vi "文本文件（将100个正弦数据以3位小数的形式写入文本文件的尾部）.vi"() -> ()   [LabVIEW 2017]
panel:
  out "写入数据":dbl[](array[numeric])
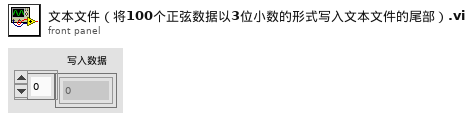
[diagram p1: front panel]
types:
  T1 = enum16{"open", "replace", "create", "open or create", "replace or create", "replace or create with confirmation"}
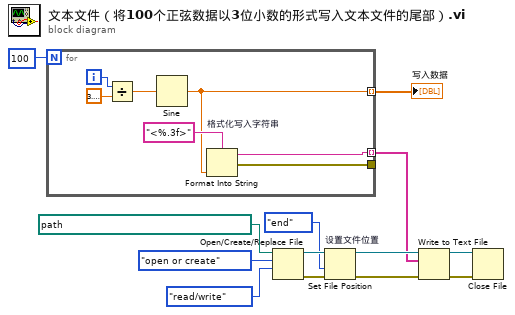
[diagram p0: block diagram]
diagram:
  n1 = for {
    N: 100 -> [_]
    tunnel: [w16] -> w3 mode=indexing
    tunnel: [w15] -> _
    tunnel: [w14] -> w12 mode=indexing
    i -> [w20]
    n2 = Divide(x=w20, y=3.141592653589793) -> (x/y=w18:dbl)
    n3 = Sine(x=w18) -> (sin(x)=w14:dbl)
    n4 = Format Into String "格式化写入字符串"(format string="<%.3f>" ("格式字符串"), w14) -> (resulting string=w16:string, error out=w15:errorcluster)  [unwired: 2 in]
  }
  "写入数据" <- w12
  n5 = Open/Create/Replace File(file path (use dialog)=path "E:/学科资料/LabView/复习/ex5-3.txt" ("文件（使用对话框）"), operation (0:open)=T1."open or create" ("操作(0:open)"), access (0:read/write)=enum16{"read/write", "read-only", "write-only"}."read/write" ("权限(0:read/write)")) -> (refnum out=w8:refnum<file>, error out=w7:errorcluster)  [unwired: 3 in, 1 out]
  n6 = Set File Position "设置文件位置"(refnum=w8, from (0:start)=enum16{"start", "end", "current"}."end" ("自（0:起始）"), error in=w7) -> (refnum out=w5:refnum<file>, error out=w4:errorcluster)  [unwired: 1 in]
  n7 = Write to Text File(file (use dialog)=w5, text=w3, error in=w4) -> (refnum out=w2:refnum<file>, error out=w1:errorcluster)  [unwired: 1 in, 1 out]
  n8 = Close File(refnum=w2, error in=w1) -> ()  [unwired: 2 out]
